vi "Card Selector.vi"(9 "# Of Cards Total":i32, 11 "Card Cluster":T1) -> (2 "Card to use":i32)   [LabVIEW 2012, in "Universal Power Meter.lvlib" / "WT1600.lvlib" / "WT1600.lvclass"]
uses:
  WT1600.lvclass
panel:
  out "Numeric":i32
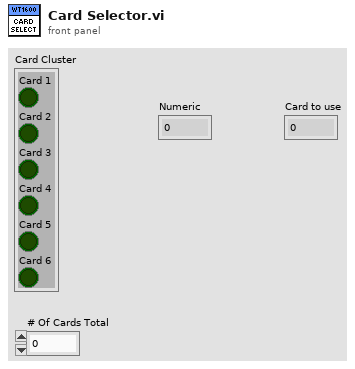
[diagram p1: front panel]
types:
  T1 = cluster{"Card 1":bool, "Card 2":bool, "Card 3":bool, "Card 4":bool, "Card 5":bool, "Card 6":bool}
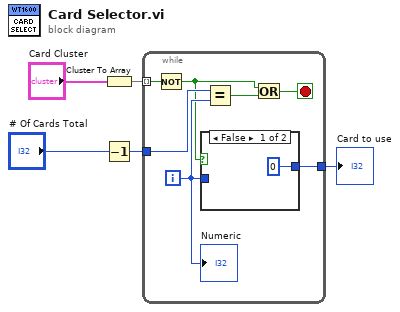
[diagram p0: block diagram]
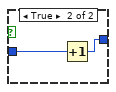
[diagram p2: hidden frame]
diagram:
  n1 = Cluster To Array(cluster="Card Cluster") -> (array=w5:bool[])
  n2 = Decrement(x="# Of Cards Total") -> (x-1=w4:i32)
  n3 = while {
    tunnel: w5 -> [w7] mode=indexing
    tunnel: w4 -> [w12]
    tunnel: [w10] -> w3
    i -> [w11]
    stop <- w8 stop-if-true
    n4 = Not(x=w7) -> (.not. x?=w6:bool)
    n5 = case shown="False" w6 {
      tunnel: w11 -> [_ w15]
      tunnel: [0 w14] -> w10
      frame False {
      }
      frame True {
        n6 = Increment(x=w15) -> (x+1=w14:i32)
      }
    }
    n7 = Equal?(x=w12, y=w11) -> (x = y?=w9:bool)
    n8 = Or(x=w6, y=w9) -> (x .or. y?=w8:bool)
    "Numeric" <- w11
  }
  "Card to use" <- w3
